vi "SynapseAPI-Get Mode (string).vi"(0 "URL":string="http://localhost:24414", 11 "error in (no error)":errorcluster) -> (8 "mode":string, 15 "error out":errorcluster)   [LabVIEW 2015]
uses:
  <vilib>/httpClient/LabVIEWHTTPClient.lvlib
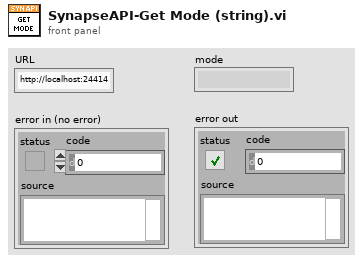
[diagram p1: front panel]
types:
  T1 = typedef "LabVIEWHTTPClient.lvlib/ClientHandle.ctl" = refnum<k1>
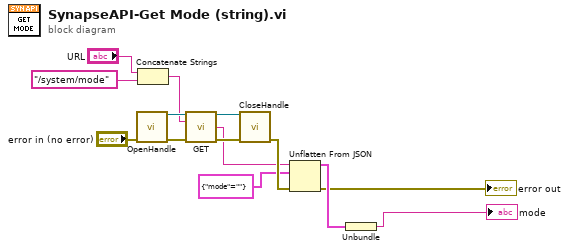
[diagram p0: block diagram]
diagram:
  n1 = call <vilib>:"OpenHandle.vi"("error in (no error)"="error in (no error)") -> ("client handle out"=w11:T1, "error out"=w10:errorcluster)  [unwired: 13 in]
  n2 = Concatenate Strings("URL", "/system/mode") -> (w3:string)
  n3 = call <vilib>:"GET.vi"("client handle"=w11, "url"=w3, "error in (no error)"=w10) -> ("client handle out"=w13:T1, "body"=w7:string, "error out"=w14:errorcluster)  [unwired: 9 in, 1 out]
  n4 = call <vilib>:"CloseHandle.vi"("client handle"=w13, "error in (no error)"=w14) -> ("error out"=w9:errorcluster)  [unwired: 13 in]
  n5 = Unflatten From JSON(JSON string=w7, type and defaults=cluster{"mode":string} {"mode"=""} ("Cluster"), error in (no error)=w9) -> (value=w5:cluster{"mode":string}, error out=→"error out":errorcluster)  [unwired: 4 in]
  n6 = Unbundle(w5) -> ("mode"=→"mode":string)
